vi "Slip_Init.vi"(0 "VISA Refnum in":refnum<visa-resource-name>="COM9", 9 "baud rate":u32=250000, 11 "error in":errorcluster) -> (4 "VISA resource name out":refnum<visa-resource-name>, 8 "NumBytesAtPort":u32, 15 "error out":errorcluster)   [LabVIEW 2020]
doc: "Starts the sync byte and initializes comms."
uses:
  SlipDataCluster.ctl
  <vilib>/Instr/_visa.llb/VISA Flush IO Buffer Mask.ctl
  <vilib>/Instr/_visa.llb/VISA Configure Serial Port (Instr).vi
panel:
  out "output cluster":T1[](array[typedef])
  out "All Strings received":string[](array[string])
  out "latest payload":T1
  in  "PacketSize(bytes)":i32=14
  in  "stop":bool
  out "Loop Error":bool
  out "last string Recvd":string
  out "Error":bool
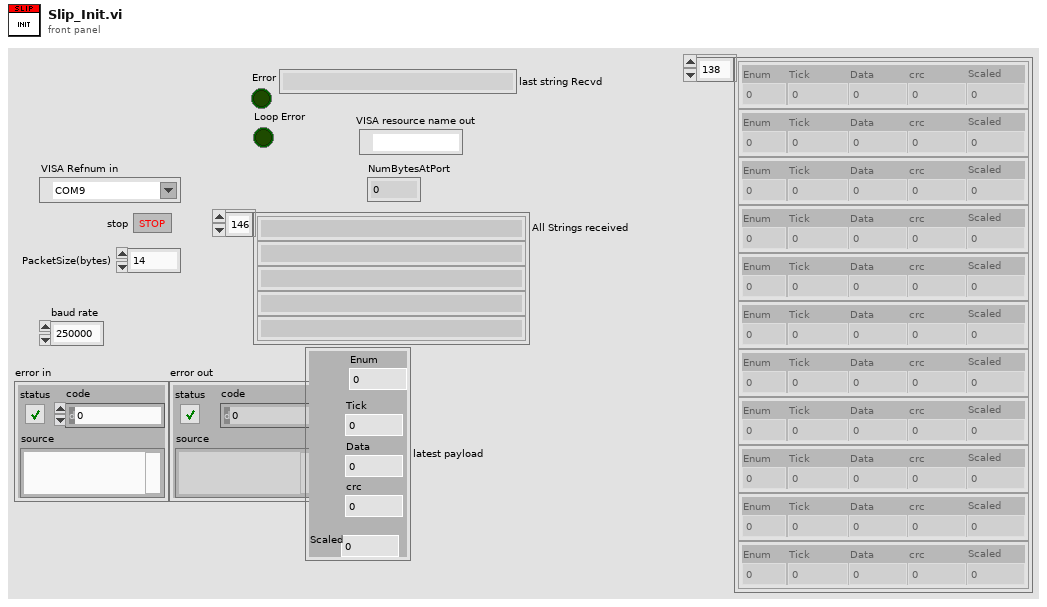
[diagram p1: front panel]
types:
  T1 = typedef "SlipDataCluster.ctl" = cluster{"Enum":u16, "Tick":u32, "Data":u32, "crc":u16, "Scaled":dbl}
  T2 = typedef "VISA Flush IO Buffer Mask.ctl" = u16
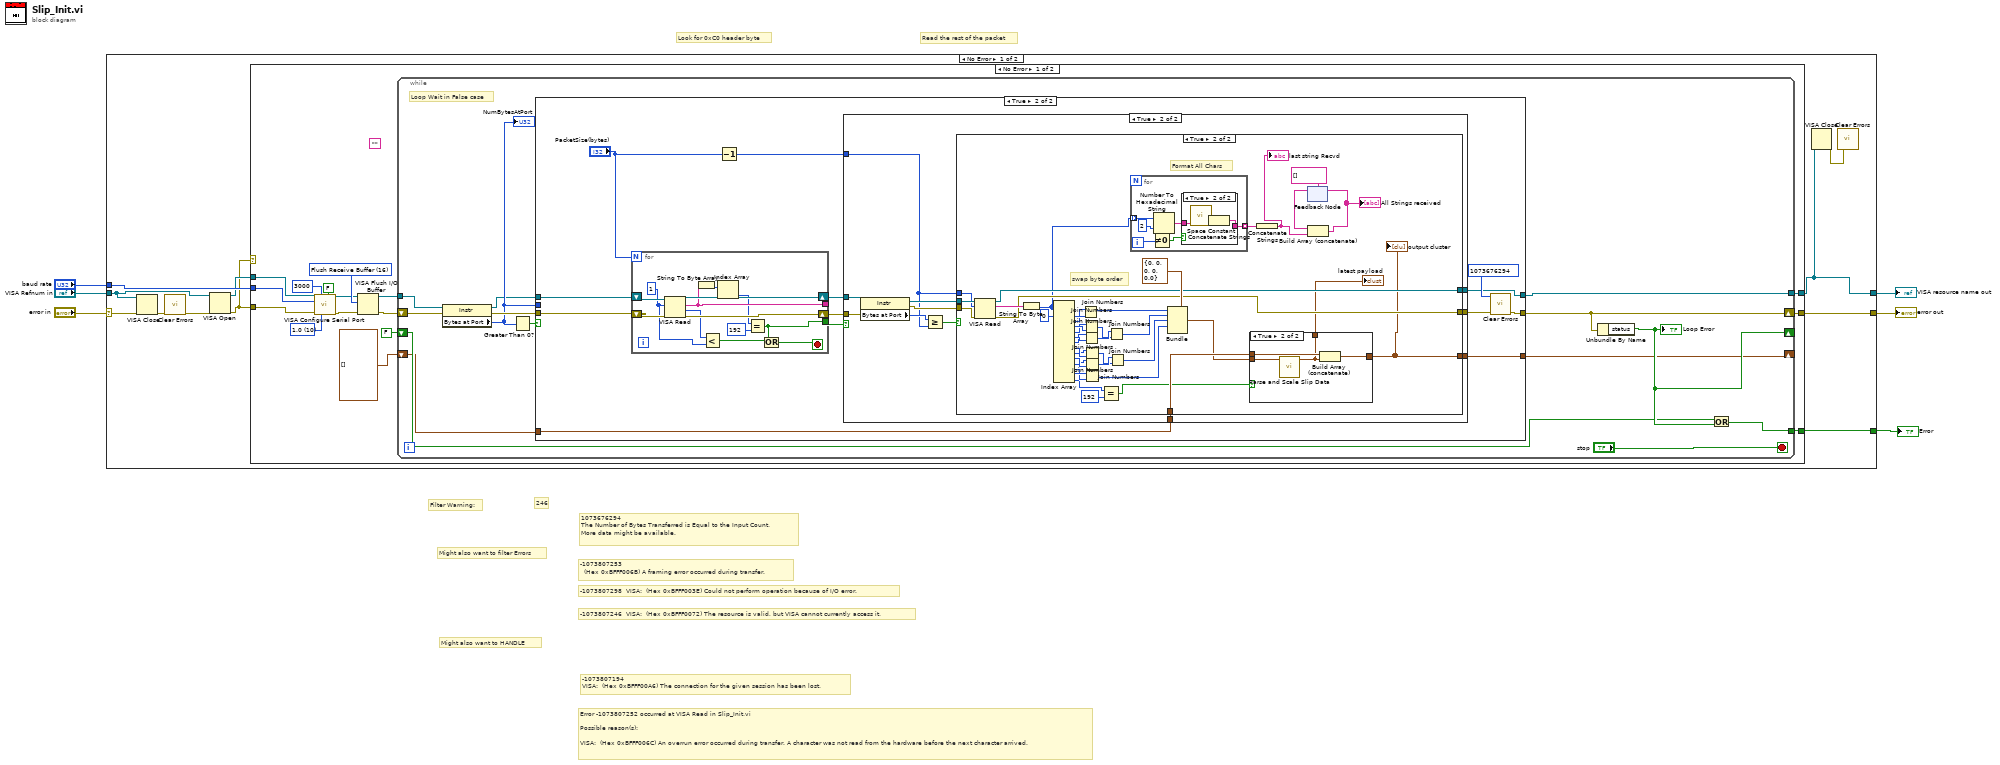
[diagram p0: block diagram]
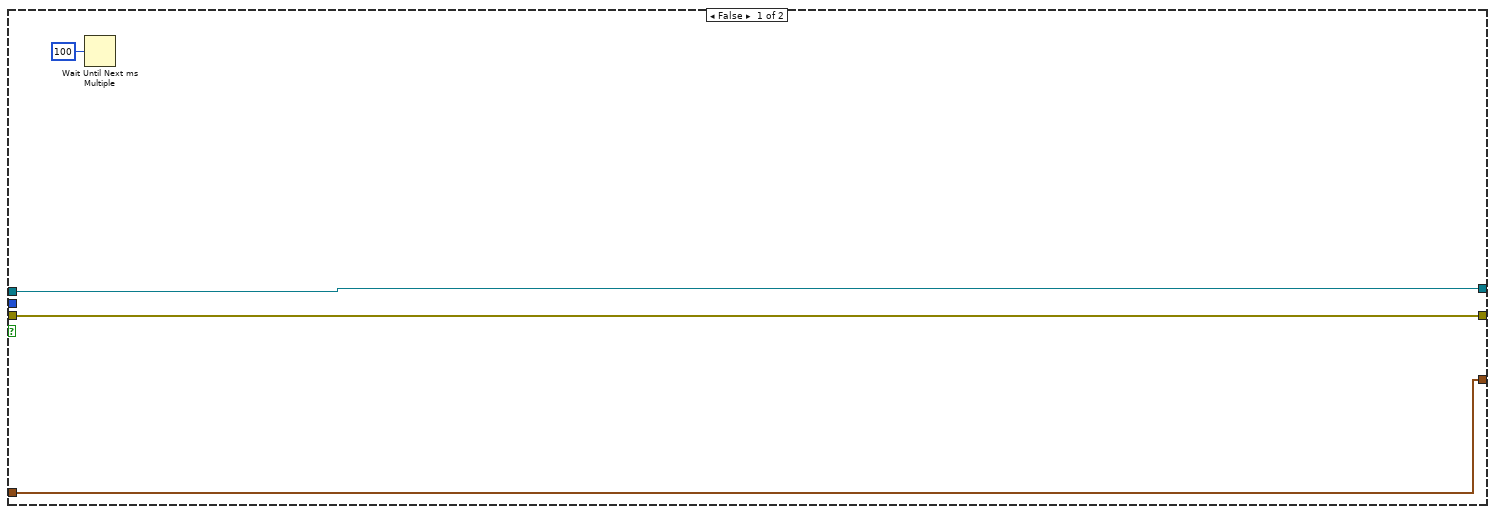
[diagram p2: hidden frame]
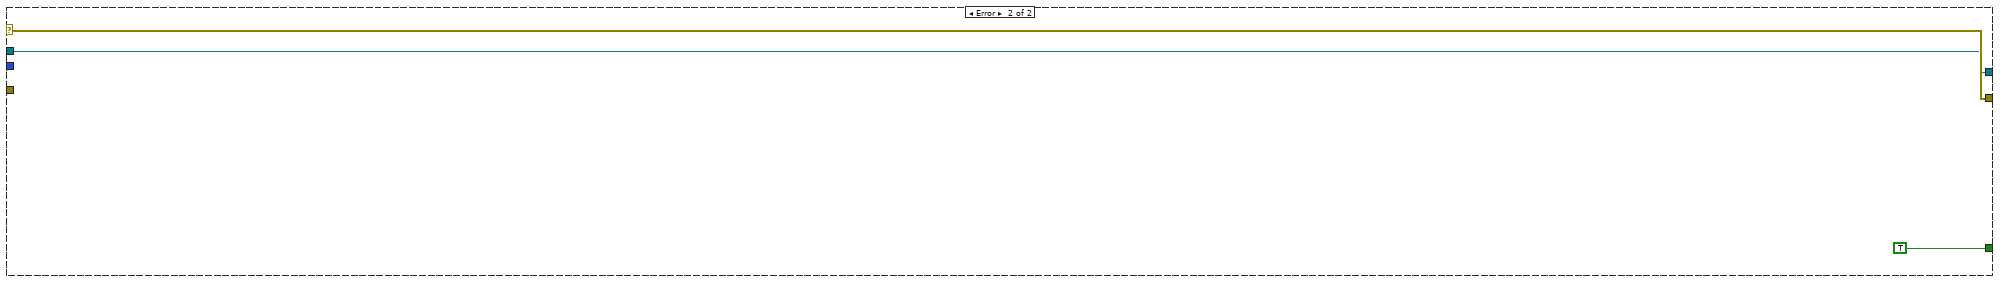
[diagram p7: hidden frame]
diagram:
  # "Error -1073807252 occurred at VISA Read in Slip_Init.vi\n\nPossible reason(s):\n\nVISA:  (Hex 0xBFFF006C) An overrun error occurred during transfer. A character was not read from the hardware before the next character arrived."
  # "Might also want to HANDLE"
  # "-1073807194\nVISA:  (Hex 0xBFFF00A6) The connection for the given session has been lost."
  # "-1073807246  VISA:  (Hex 0xBFFF0072) The resource is valid, but VISA cannot currently access it."
  # "246"
  # "Read the rest of the packet"
  # "Look for 0xC0 header byte"
  # "Filter Warning:"
  # "Might also want to filter Errors"
  # "-1073807298  VISA:  (Hex 0xBFFF003E) Could not perform operation because of I/O error."
  # "-1073807253\n  (Hex 0xBFFF006B) A framing error occurred during transfer."
  # "1073676294\nThe Number of Bytes Transferred is Equal to the Input Count. \nMore data might be available."
  n1 = case shown="No Error" "error in" {
    selector: "error in" -> [w14 w155]
    tunnel: [w17 w155] -> w6
    tunnel: "baud rate" -> [w16 _]
    tunnel: [w11 w154] -> w4
    tunnel: "VISA Refnum in" -> [w15 w154]
    tunnel: [w13 _] -> w1
    frame No Error {
      n2 = VISA Close(VISA resource name=w15, error in (no error)=w14) -> (error out=w12:errorcluster)
      n3 = call <vilib>:"Clear Errors.vi"("error in (no error)"=w12) -> ("error out"=w9:errorcluster)  [unwired: 5 in, 1 out]
      n4 = VISA Open(error in (no error)=w9, VISA resource name=w15) -> (VISA resource name=w8:refnum<visa-resource-name>, error out=w7:errorcluster)  [unwired: 3 in]
      n5 = case shown="No Error" w7 {
        selector: w7 -> [_ w153]
        tunnel: [w33 w153] -> w17
        tunnel: w16 -> [w32 _]
        tunnel: [w26 TRUE] -> w13
        tunnel: [w22 w152] -> w11
        tunnel: w7 -> [w19 _]
        tunnel: w8 -> [w18 w152]
        frame No Error {
          (unwired) ""
          w30 = T2 16 items=["Flush Receive Buffer"=16, "Write Transmit Buffer to Device"=32, "Flush Receive Buffer (No I/O)"=64, "Flush Transmit Buffer"=128] ("Mask")
          w31 = u16 10 items=["1.0"=10, "1.5"=15, "2.0"=20] ("stop bits (10: 1 bit)")
          n6 = call-poly "VISA Configure Serial Port"("VISA resource name"=w18, "timeout (10sec)"=u32 3000, "Enable Termination\nChar (T)"=FALSE ("Enable Termination\nChar (T)"), "baud rate (9600)"=w32, "error in (no error)"=w19, "stop bits (10: 1 bit)"=w31) -> ("VISA resource name out"=w28:refnum<visa-resource-name>, "error out"=w27:errorcluster)  [unwired: 8 in]
          n7 = VISA Flush I/O Buffer(VISA resource name=w28, mask (16)=w30, error in (no error)=w27) -> (VISA resource name out=w24:refnum<visa-resource-name>, error out=w25:errorcluster)
          n8 = while {
            tunnel: [w43] -> w22
            tunnel: [w37] -> w26
            shift-right: [w39] -> w33
            shift-left: w25 -> [w42]
            tunnel: w24 -> [w40]
            shift-right: [w38] -> _
            shift-left: FALSE ("status") -> [w36]
            shift-right: [w35] -> _
            shift-left: T1[] [] -> [w34]
            stop <- "stop" stop-if-true
            # "Loop Wait in False case"
            n9 = property class="Instr"(reference=w40, error in=w42) -> (reference out=w44:refnum<visa-resource-name>, error out=w47:errorcluster, "Bytes at Port"=w46:u32)
            "NumBytesAtPort" <- w46
            n10 = Greater Than 0?(x=w46) -> (x > 0?=w45:bool)
            n11 = case shown="True" w45 {
              tunnel: w44 -> [w50 w64]
              tunnel: w46 -> [_ _]
              tunnel: w47 -> [w51 w63]
              tunnel: [w51 w61] -> w39
              tunnel: [w50 w53] -> w43
              tunnel: [w49 w55] -> w35
              tunnel: w34 -> [w49 w54]
              frame False {
                n12 = Wait Until Next ms Multiple(millisecond multiple=u32 100) -> ()  [unwired: 1 out]
              }
              frame True {
                n13 = for {
                  N: "PacketSize(bytes)" -> [_]
                  tunnel: [w146] -> _
                  shift-right: [w148] -> w59
                  shift-left: w64 -> [w150]
                  shift-right: [w147] -> w58
                  shift-left: w63 -> [w149]
                  tunnel: [w139] -> w60
                  stop <- w138 stop-if-true
                  w141 = u32 1 ("byte count")
                  n14 = VISA Read(VISA resource name=w150, byte count=w141, error in (no error)=w149) -> (VISA resource name out=w148:refnum<visa-resource-name>, read buffer=w146:string, return count=w142:u32, error out=w147:errorcluster)
                  n15 = String To Byte Array(string=w146) -> (unsigned byte array=w145:u8[])
                  n16 = Less?(x=w142, y=w141) -> (x < y?=w140:bool)
                  n17 = Index Array(array=w145) -> (element=w144:u8)  [unwired: 1 in]
                  n18 = Equal?(x=w144, y=u8 192) -> (x = y?=w139:bool)
                  n19 = Or(x=w139, y=w140) -> (x .or. y?=w138:bool)
                }
                n20 = Decrement(x="PacketSize(bytes)") -> (x-1=w56:i32)
                n21 = case shown="True" w60 {
                  tunnel: w59 -> [w66 w78]
                  tunnel: w58 -> [w65 w77]
                  tunnel: w56 -> [_ w72]
                  tunnel: [w67 w71] -> w55
                  tunnel: w54 -> [w67 w70]
                  tunnel: [w66 w69] -> w53
                  tunnel: [w65 w68] -> w52
                  frame False {
                  }
                  frame True {
                    n22 = property class="Instr"(reference=w78, error in=w77) -> (reference out=w74:refnum<visa-resource-name>, error out=w73:errorcluster, "Bytes at Port"=w76:u32)
                    n23 = Greater Or Equal?(x=w76, y=w72) -> (x >= y?=w75:bool)
                    n24 = case shown="True" w75 {
                      tunnel: w74 -> [w81 w122]
                      tunnel: w73 -> [w80 w121]
                      tunnel: w72 -> [_ w119]
                      tunnel: [w79 w82] -> w71
                      tunnel: w70 -> [w79 w94]
                      tunnel: [w81 w93] -> w69
                      tunnel: [w80 w92] -> w68
                      frame False {
                      }
                      frame True {
                        # "Format All Chars"
                        # "swap byte order"
                        n25 = VISA Read(VISA resource name=w122, byte count=w119, error in (no error)=w121) -> (VISA resource name out=w93:refnum<visa-resource-name>, read buffer=w120:string, error out=w92:errorcluster)  [unwired: 1 out]
                        n26 = String To Byte Array(string=w120) -> (unsigned byte array=w91:u8[])
                        n27 = Index Array(array=w91, index #1=0 ("index")) -> (element #1=w117:u8, element #2=w116:u8, element #3=w114:u8, element #4=w113:u8, element #5=w112:u8, element #6=w111:u8, element #7=w105:u8, element #8=w104:u8, element #9=w103:u8, element #10=w102:u8, element #11=w99:u8, element #12=w100:u8, element #13=w96:u8)  [unwired: 12 in]
                        n28 = Join Numbers(hi=w116, lo=w117) -> ((hi.lo)=w115:u16)
                        n29 = Join Numbers(hi=w113, lo=w114) -> ((hi.lo)=w109:u16)
                        n30 = Join Numbers(hi=w111, lo=w112) -> ((hi.lo)=w110:u16)
                        n31 = Join Numbers(hi=w104, lo=w105) -> ((hi.lo)=w106:u16)
                        n32 = Join Numbers(hi=w102, lo=w103) -> ((hi.lo)=w107:u16)
                        n33 = Join Numbers(hi=w100, lo=w99) -> ((hi.lo)=w98:u16)
                        n34 = Equal?(x=w96, y=u8 192) -> (x = y?=w83:bool)
                        n35 = Join Numbers(hi=w110, lo=w109) -> ((hi.lo)=w108:u32)
                        n36 = Join Numbers(hi=w107, lo=w106) -> ((hi.lo)=w101:u32)
                        n37 = for {
                          tunnel: w91 -> [w131] mode=indexing
                          tunnel: [w130] -> w90 mode=indexing
                          i -> [w129]
                          n38 = Not Equal To 0?(x=w129) -> (x != 0?=w128:bool)
                          n39 = Number To Hexadecimal String(1:i16 2 ("width (-)"), 2:w131) -> (0:w133:string)
                          n40 = case shown="True" w128 {
                            tunnel: w133 -> [w134 w137]
                            tunnel: [w134 w136] -> w130
                            frame False {
                            }
                            frame True {
                              n41 = call <vilib>:"Space Constant.vi"() -> ("String"=w135:string)
                              n42 = Concatenate Strings(w135, w137) -> (w136:string)
                            }
                          }
                        }
                        n43 = Bundle(cluster=T1 {"Enum"=0, "Tick"=0, "Data"=0, "crc"=0, "Scaled"=0.0} ("output cluster"), "Enum"=w115, "Tick"=w108, "Data"=w101, "crc"=w98) -> (w85:T1)  [unwired: 1 in]
                        n44 = case shown="True" w83 {
                          tunnel: [w123 w127] -> w82
                          tunnel: w94 -> [w123 w126]
                          tunnel: w85 -> [_ w125]
                          tunnel: [_ w124] -> w84
                          frame False {
                            # "bad footer"
                          }
                          frame True {
                            n45 = call "Parse and Scale Slip Data.vi"("Slip cluster In"=w125) -> ("Slip Cluster Out"=w124:T1)  [unwired: 10 in]
                            n46 = Build Array (concatenate)(w126, w124) -> (w127:T1[])
                          }
                        }
                        "latest payload" <- w84
                        "output cluster" <- w82
                        n47 = Concatenate Strings(w90) -> (w89:string)
                        "last string Recvd" <- w89
                        n48 = feedback #1(string[] []) -> (w87:string[])
                        n49 = Build Array (concatenate)(w87, w89) -> (w88:string[])
                        "All Strings received" <- w88
                        n50 = feedback-in #1(w88) -> ()
                      }
                    }
                  }
                }
                n51 = call <vilib>:"Clear Errors.vi"("error in (no error)"=w52, "specific error code to clear (0: all)"=1073676294) -> ("error out"=w61:errorcluster)  [unwired: 4 in, 1 out]
              }
            }
            n52 = Unbundle By Name(w39) -> ("status"=w38:bool)
            "Loop Error" <- w38
            n53 = Or(x=w36, y=w38) -> (x .or. y?=w37:bool)
          }
        }
        frame Error {
        }
      }
      n54 = VISA Close(VISA resource name=w11) -> (error out=w10:errorcluster)  [unwired: 1 in]
      n55 = call <vilib>:"Clear Errors.vi"("error in (no error)"=w10) -> ()  [unwired: 5 in, 2 out]
    }
    frame Error {
    }
  }
  "error out" <- w6
  "VISA resource name out" <- w4
  "Error" <- w1
